vi "Get_Error_Status.vi"(5 "Device Number":T1, 7 "Update":bool, 8 "error in":errorcluster) -> (0 "error out":errorcluster)   [LabVIEW 2016]
doc: "This navX VI returns the velocity and displacement of the navX. This VI is only supported on firmware virsions newer than 2.2.xxx."
uses:
  TypeDefs/FRIC_navX_DeviceNumbersTypeDef.ctl
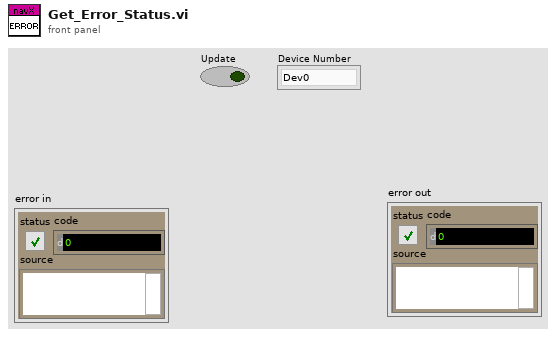
[diagram p1: front panel]
types:
  T1 = typedef "FRIC_navX_DeviceNumbersTypeDef.ctl" = enum16{"Dev0", "Dev1", "Dev2", "Dev3"}
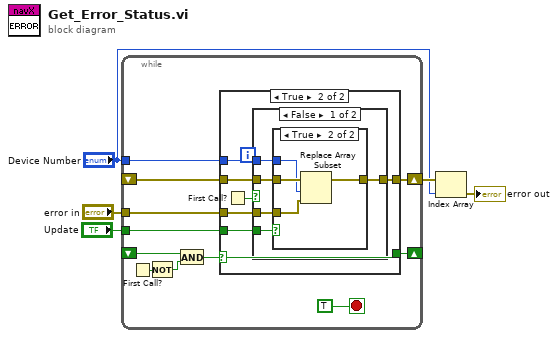
[diagram p0: block diagram]
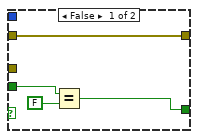
[diagram p2: hidden frame]
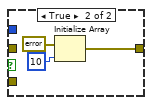
[diagram p4: hidden frame]
diagram:
  n1 = while {
    shift-right: [w16] -> w4
    shift-left: _ -> [w14]
    tunnel: "Update" -> [w13]
    tunnel: "Device Number" -> [w12]
    tunnel: "error in" -> [w11]
    shift-right: [w6] -> _
    shift-left: _ -> [w8]
    stop <- TRUE stop-if-true
    n2 = First Call?() -> (First Call?: T/F=w10:bool)
    n3 = Not(x=w10) -> (.not. x?=w9:bool)
    n4 = And(x=w8, y=w9) -> (x .and. y?=w7:bool)
    n5 = case shown="True" w7 {
      selector: w7 -> [_ w21]
      tunnel: [w20 w27] -> w16
      tunnel: w14 -> [w20 w26]
      tunnel: w13 -> [w18 w25]
      tunnel: w12 -> [_ w24]
      tunnel: w11 -> [_ w23]
      tunnel: [w17 w21] -> w6
      frame False {
        n6 = Equal?(x=w18, y=FALSE) -> (x = y?=w17:bool)
      }
      frame True {
        n7 = First Call?() -> (First Call?: T/F=w22:bool)
        n8 = case shown="False" w22 {
          tunnel: [w32 w39] -> w27
          tunnel: w26 -> [w31 _]
          tunnel: w25 -> [w29 _]
          tunnel: w24 -> [w30 _]
          tunnel: w23 -> [w28 _]
          frame False {
            n9 = case shown="True" w29 {
              tunnel: [w33 w36] -> w32
              tunnel: w31 -> [w33 w37]
              tunnel: w30 -> [_ w35]
              tunnel: w28 -> [_ w34]
              frame False {
              }
              frame True {
                n10 = Replace Array Subset(array=w37, new element=w34, index=w35) -> (w36:errorcluster[])
              }
            }
          }
          frame True {
            n11 = Initialize Array(errorcluster {"status"=FALSE, "code"=0, "source"=""} ("error"), 10 ("dimension size")) -> (w39:errorcluster[])
          }
        }
      }
    }
  }
  n12 = Index Array(array=w4, index="Device Number") -> (element=→"error out":errorcluster)
